vi "Save data to file (string).vi"(8 "File path":path, 9 "Save data?":bool, 11 "Data":string[](array[string])) -> ()   [LabVIEW 2018]
uses:
  <vilib>/Utility/file.llb/Write Delimited Spreadsheet (string).vi
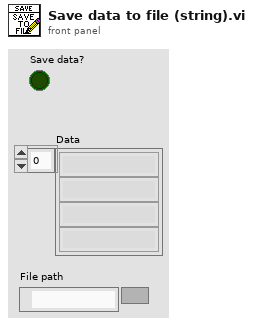
[diagram p1: front panel]
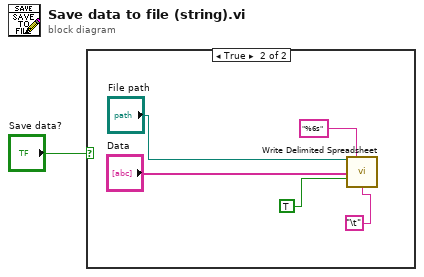
[diagram p0: block diagram]
diagram:
  n1 = case shown="True" "Save data?" {
    frame False {
    }
    frame True {
      n2 = call-poly <vilib>:"Write Delimited Spreadsheet.vi"("file path (dialog if empty)"="File path", "format (%s)"="%6s" ("format (%.3f)"), "1D data"="Data", "append to file? (new file:F)"=TRUE, "delimiter (\\t)"="\t") -> ()  [unwired: 9 in, 2 out]
    }
  }
